vi "Signal-cameravision.vi"(7 "Vision action":T1=enum."Start", 8 "error in (no error)":errorcluster, 11 "Object ref in":T2) -> (0 "error out":errorcluster, 3 "Object ref out":T2)   [LabVIEW 2013, in "SLMControl.lvlib" / "SC-Main.lvclass"]
uses:
  SC-Main.lvclass
  Object-reference.ctl
  Vision-actions.ctl
  SC-Main.lvclass/SC-Main.ctl
  Client/Sources/Supported-modules.ctl
  Read Client.vi
  Read CameraVision.vi
  Client/Sources/SC-Client.lvclass
  SA-SLMAPI/Sources/Action/Action.lvclass
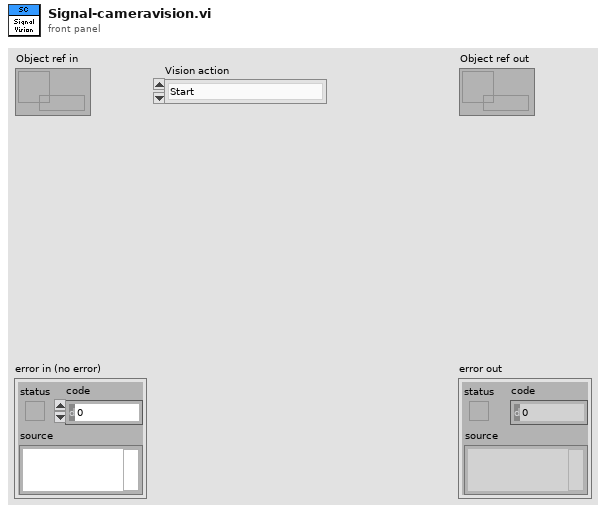
[diagram p1: front panel]
types:
  T1 = typedef "SLMControl.lvlib/SC-Main.lvclass/Vision-actions.ctl" = enum16{"Activate", "Start", "Repeat", "Stop", "Exit"}
  T2 = typedef "SLMControl.lvlib/SC-Main.lvclass/Object-reference.ctl" = refnum<data-value>
  T3 = typedef "SLMControl.lvlib/SC-Client.lvclass/Object-reference.ctl" = refnum<data-value>
  T4 = typedef "SLMControl.lvlib/SC-Client.lvclass/Supported-modules.ctl" = enum16{"Server", "All", "SLMControl", "PowderDeposition", "StrategyParser", "CameraVision", "MaterialCharacterization", "StatusMonitor", "SLMSimulation", "LaserCharacterization"}
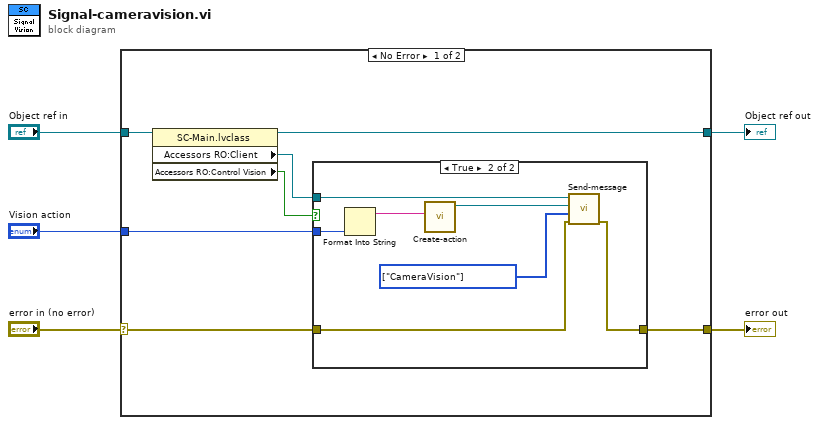
[diagram p0: block diagram]
diagram:
  n1 = case shown="No Error" "error in (no error)" {
    selector: "error in (no error)" -> [w8 w22]
    tunnel: [w7 w22] -> w4
    tunnel: [w11 w21] -> w2
    tunnel: "Object ref in" -> [w12 w21]
    tunnel: "Vision action" -> [w10 _]
    frame No Error {
      n2 = property class="SC-Main.lvclass"(reference=w12) -> (reference out=w11:T2, "Accessors RO:Client"=w9:T3, "Accessors RO:Control Vision"=w6:bool)  [unwired: 1 in, 1 out]
      n3 = case shown="True" w6 {
        tunnel: w10 -> [_ w20]
        tunnel: w9 -> [_ w18]
        tunnel: w8 -> [w13 w16]
        tunnel: [w13 w15] -> w7
        frame False {
        }
        frame True {
          w14 = T4[] [enum."CameraVision"] items=["Server", "All", "SLMControl", "PowderDeposition", "StrategyParser", "CameraVision", "MaterialCharacterization", "StatusMonitor", "SLMSimulation", "LaserCharacterization"] ("Receivers")
          n4 = Format Into String(w20) -> (resulting string=w19:string)  [unwired: 3 in, 1 out]
          n5 = call "Create-action.vi"("Action"=w19) -> ("Action out"=w17:refnum<class "Action.lvclass">)  [unwired: 9 in, 1 out]
          n6 = call "Send-message.vi"("error in (no error)"=w16, "Receivers"=w14, "Message"=w17, "Client in"=w18) -> ("error out"=w15:errorcluster)  [unwired: 6 in, 1 out]
        }
      }
    }
    frame Error {
    }
  }
  "error out" <- w4
  "Object ref out" <- w2
